vi "ViperHawk Check and Filter Inv Data.vi"(7 "Enum":enum16{"Inv Data", "MC Data"}(ring), 11 "Diagnostic Data In":T1) -> (3 "Diagnostic Data Out":T1)   [LabVIEW 2016]
uses:
  Type Definitions/ViperHawk/ViperHawk Diagnostic Data.ctl
  <vilib>/ptbypt/NI_PtbyPt.lvlib
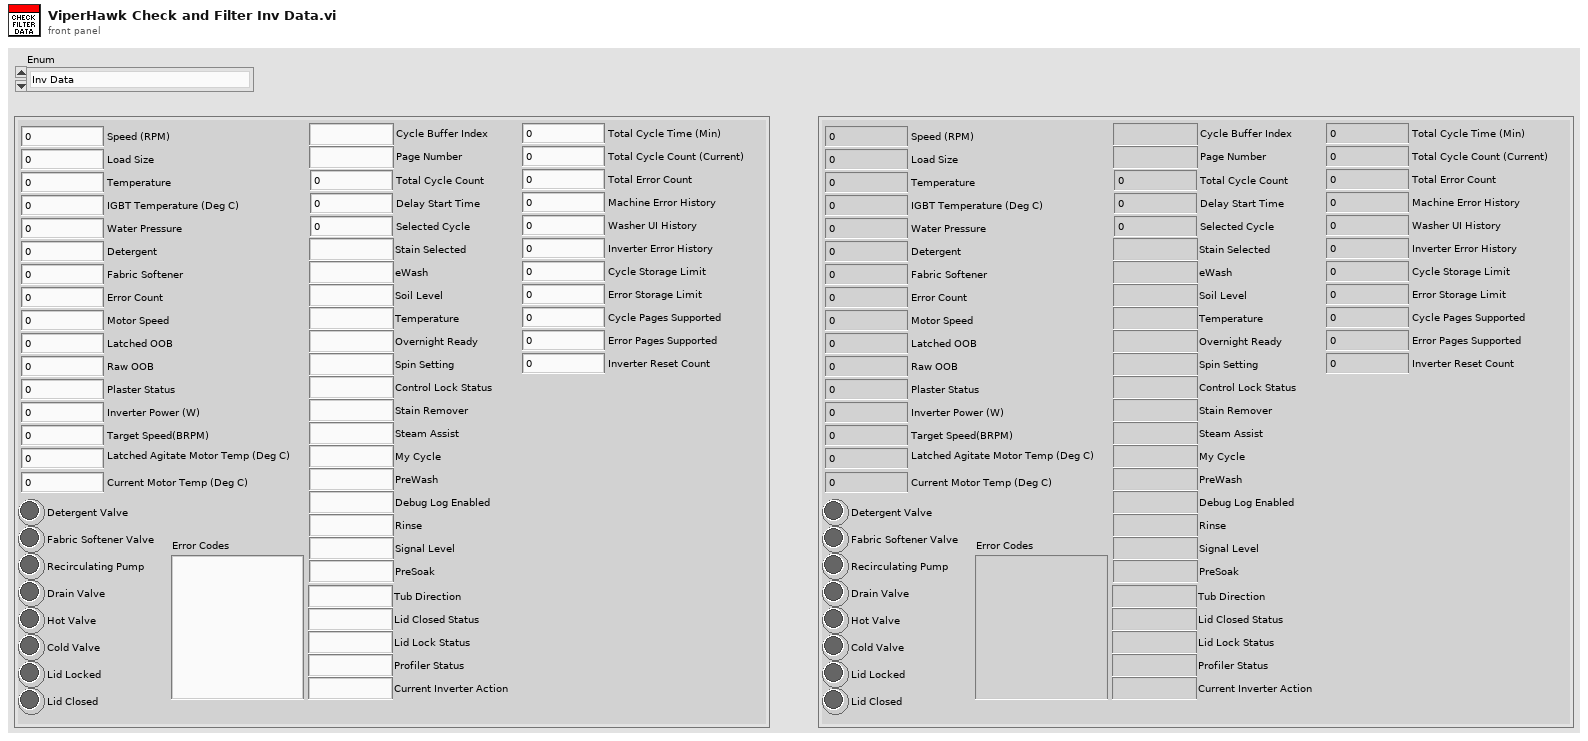
[diagram p1: front panel]
types:
  T1 = typedef "ViperHawk Diagnostic Data.ctl" = cluster{"Speed (RPM)":u32, "Load Size":u32, "Temperature":u32, "Water Pressure":dbl, "Detergent":u32, "Fabric Softener":u32, "Tub Direction":string, "Detergent Valve":bool, "Fabric Softener Valve":bool, "Recirculating Pump":bool, "Drain Valve":bool, "Hot Valve":bool, "Cold Valve":bool, "Lid Closed Status":string, "Lid Lock Status":string, "Error Count":u32, "IGBT Temperature (Deg C)":u32, "Motor Speed":u32, "Latched OOB":u32, "Raw OOB":u32, "Plaster Status":u32, "Inverter Power (W)":u32, "Target Speed(BRPM)":u32, "Latched Agitate Motor Temp (Deg C)":u32, "Current Motor Temp (Deg C)":u32, "Profiler Status":string, "Current Inverter Action":string, "Error Codes":string, "Lid Locked":bool, "Lid Closed":bool, "9E Diagnostic Data":cluster{"Total Cycle Time (Min)":u32, "Total Cycle Count (Current)":u16, "Total Error Count":u16, "Machine Error History":u32, "Washer UI History":u32, "Inverter Error History":u32, "Cycle Storage Limit":u8, "Error Storage Limit":u8, "Cycle Pages Supported":u8, "Error Pages Supported":u8, "Inverter Reset Count":u16}, "9F Diagnostic Data":cluster{"Cycle Buffer Index":string, "Page Number":string, "Total Cycle Count":u32, "Delay Start Time":u32, "Stain Selected":string, "Selected Cycle":u32, "eWash":string, "Soil Level":string, "Temperature":string, "Overnight Ready":string, "Spin Setting":string, "Control Lock Status":string, "Stain Remover":string, "Steam Assist":string, "My Cycle":string, "PreWash":string, "Debug Log Enabled":string, "Rinse":string, "Signal Level":string, "PreSoak":string}}
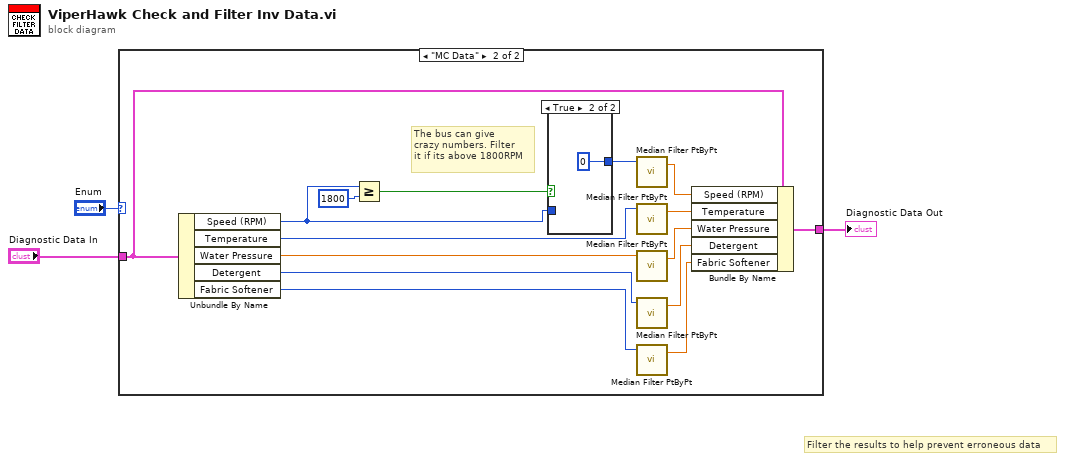
[diagram p0: block diagram]
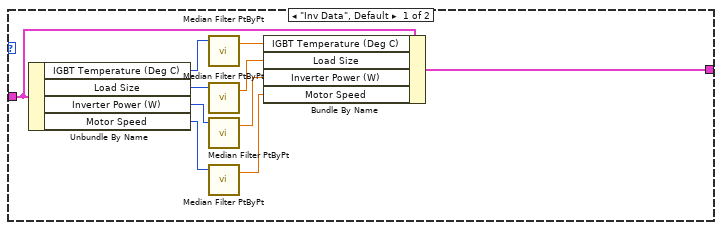
[diagram p2: hidden frame]
diagram:
  # "Filter the results to help prevent erroneous data"
  n1 = case shown="\"MC Data\"" "Enum" {
    tunnel: "Diagnostic Data In" -> [w12 w28]
    tunnel: [w13 w27] -> w1
    frame "Inv Data", Default {
      n2 = Unbundle By Name(w12) -> ("IGBT Temperature (Deg C)"=w11:u32, "Load Size"=w10:u32, "Inverter Power (W)"=w7:u32, "Motor Speed"=w6:u32)
      n3 = call <vilib>:"Median Filter PtByPt.vi"("x"=w11) -> ("Filtered x"=w8:dbl)  [unwired: 3 in, 1 out]
      n4 = call <vilib>:"Median Filter PtByPt.vi"("x"=w10) -> ("Filtered x"=w9:dbl)  [unwired: 3 in, 1 out]
      n5 = call <vilib>:"Median Filter PtByPt.vi"("x"=w7) -> ("Filtered x"=w5:dbl)  [unwired: 3 in, 1 out]
      n6 = call <vilib>:"Median Filter PtByPt.vi"("x"=w6) -> ("Filtered x"=w4:dbl)  [unwired: 3 in, 1 out]
      n7 = Bundle By Name(cluster=w12, "IGBT Temperature (Deg C)"=w8, "Load Size"=w9, "Inverter Power (W)"=w5, "Motor Speed"=w4) -> (w13:T1)
    }
    frame "MC Data" {
      # "The bus can give\ncrazy numbers. Filter\nit if its above 1800RPM"
      n8 = Unbundle By Name(w28) -> ("Speed (RPM)"=w17:u32, "Temperature"=w14:u32, "Water Pressure"=w25:dbl, "Detergent"=w23:u32, "Fabric Softener"=w21:u32)
      n9 = Greater Or Equal?(x=w17, y=u32 1800) -> (x >= y?=w18:bool)
      n10 = case shown="True" w18 {
        tunnel: [w29 u32 0 ("Speed")] -> w16
        tunnel: w17 -> [w29 _]
        frame False {
        }
        frame True {
        }
      }
      n11 = call <vilib>:"Median Filter PtByPt.vi"("x"=w16) -> ("Filtered x"=w26:dbl)  [unwired: 3 in, 1 out]
      n12 = call <vilib>:"Median Filter PtByPt.vi"("x"=w14) -> ("Filtered x"=w15:dbl)  [unwired: 3 in, 1 out]
      n13 = call <vilib>:"Median Filter PtByPt.vi"("x"=w25) -> ("Filtered x"=w24:dbl)  [unwired: 3 in, 1 out]
      n14 = call <vilib>:"Median Filter PtByPt.vi"("x"=w23) -> ("Filtered x"=w22:dbl)  [unwired: 3 in, 1 out]
      n15 = call <vilib>:"Median Filter PtByPt.vi"("x"=w21) -> ("Filtered x"=w20:dbl)  [unwired: 3 in, 1 out]
      n16 = Bundle By Name(cluster=w28, "Speed (RPM)"=w26, "Temperature"=w15, "Water Pressure"=w24, "Detergent"=w22, "Fabric Softener"=w20) -> (w27:T1)
    }
  }
  "Diagnostic Data Out" <- w1
